vi "rsidr_core_global.vi"() -> ()   [LabVIEW 2015, in "Rohde&Schwarz CMXP GPRF.lvlib"] (continued)
 All", "Data Type"=6, "Command"="FETC:GPRF:MEAS{instance}:POW:STAT:ALL?", "Access"=0, "Range Table"="", "Read Callback"="", "Write Callback"="", "Supported Models"="", "Instrument Options"="", "Flags"=0, "Help"="Queries the main measurement state and the measurement substates. Both measurement substates are relevant for running measurements only.\n\nAvailable Repeated Capabilities:\ninstance: i0, i1, i2, i3, i4, i5, i6, i7, i8, i9, i10, i11, i12, i13, i14, i15, i16, i17, i18, i19, i20, i21, i22, i23, i24, i25, i26, i27, i28, i29, i30, i31, i32\r\n\nRemote-control command(s):\nFETCh:GPRF:MEAS<i>:POWer:STATe:ALL?"}, {"Level"=3, "Class Only"=FALSE, "Identifier"="RSCMXPGPRF_ATTR_POWER_MEASUREMENT_ELAPSED_INTERVALS", "Descriptive Name"="Power Measurement Elapsed Intervals", "Data Type"=6, "Command"="FETC:GPRF:MEAS{instance}:POW:EST?", "Access"=0, "Range Table"="", "Read Callback"="", "Write Callback"="", "Supported Models"="", "Instrument Options"="", "Flags"=0, "Help"="Returns the reliability indicator and the number of elapsed measurement intervals.\n\nAvailable Repeated Capabilities:\ninstance: i0, i1, i2, i3, i4, i5, i6, i7, i8, i9, i10, i11, i12, i13, i14, i15, i16, i17, i18, i19, i20, i21, i22, i23, i24, i25, i26, i27, i28, i29, i30, i31, i32\r\n\nRemote-control command(s):\nFETCh:GPRF:MEAS<i>:POWer:ESTatistics?"}, {"Level"=2, "Class Only"=TRUE, "Identifier"="", "Descriptive Name"="Results", "Data Type"=0, "Command"="", "Access"=0, "Range Table"="", "Read Callback"="", "Write Callback"="", "Supported Models"="", "Instrument Options"="", "Flags"=0, "Help"="Power measurement results."}, {"Level"=3, "Class Only"=FALSE, "Identifier"="RSCMXPGPRF_ATTR_POWER_MEASUREMENT_POWER_CURRENT", "Descriptive Name"="Power Measurement Power Current", "Data Type"=6, "Command"="CALC:GPRF:MEAS{instance}:POW:CURR?", "Access"=0, "Range Table"="", "Read Callback"="", "Write Callback"="", "Supported Models"="", "Instrument Options"="", "Flags"=0, "Help"="Returns results for the Power mode.\n\nAvailable Repeated Capabilities:\ninstance: i0, i1, i2, i3, i4, i5, i6, i7, i8, i9, i10, i11, i12, i13, i14, i15, i16, i17, i18, i19, i20, i21, i22, i23, i24, i25, i26, i27, i28, i29, i30, i31, i32\r\n\nRemote-control command(s):\nCALCulate:GPRF:MEAS<i>:POWer:CURRent?"}, {"Level"=3, "Class Only"=FALSE, "Identifier"="RSCMXPGPRF_ATTR_FETCH_POWER_MEASUREMENT_POWER_CURRENT", "Descriptive Name"="Fetch Power Measurement Power Current", "Data Type"=6, "Command"="FETC:GPRF:MEAS{instance}:POW:CURR?", "Access"=0, "Range Table"="", "Read Callback"="", "Write Callback"="", "Supported Models"="", "Instrument Options"="", "Flags"=0, "Help"="Returns results for the Power mode.\n\nAvailable Repeated Capabilities:\ninstance: i0, i1, i2, i3, i4, i5, i6, i7, i8, i9, i10, i11, i12, i13, i14, i15, i16, i17, i18, i19, i20, i21, i22, i23, i24, i25, i26, i27, i28, i29, i30, i31, i32\r\n\nRemote-control command(s):\nFETCh:GPRF:MEAS<i>:POWer:CURRent?"}, {"Level"=3, "Class Only"=FALSE, "Identifier"="RSCMXPGPRF_ATTR_READ_POWER_MEASUREMENT_POWER_CURRENT", "Descriptive Name"="Read Power Measurement Power Current", "Data Type"=6, "Command"="READ:GPRF:MEAS{instance}:POW:CURR?", "Access"=0, "Range Table"="", "Read Callback"="", "Write Callback"="", "Supported Models"="", "Instrument Options"="", "Flags"=0, "Help"="Returns results for the Power mode.\n\nAvailable Repeated Capabilities:\ninstance: i0, i1, i2, i3, i4, i5, i6, i7, i8, i9, i10, i11, i12, i13, i14, i15, i16, i17, i18, i19, i20, i21, i22, i23, i24, i25, i26, i27, i28, i29, i30, i31, i32\r\n\nRemote-control command(s):\nREAD:GPRF:MEAS<i>:POWer:CURRent?"}, {"Level"=3, "Class Only"=FALSE, "Identifier"="RSCMXPGPRF_ATTR_READ_POWER_MEASUREMENT_POWER_AVERAGE", "Descriptive Name"="Read Power Measurement Power Average", "Data Type"=6, "Command"="READ:GPRF:MEAS{instance}:POW:AVER?", "Access"=0, "Range Table"="", "Read Callback"="", "Write Callback"="", "Supported Models"="", "Instrument Options"="", "Flags"=0, "Help"="Returns results for the Power mode.\n\nAvailable Repeated Capabilities:\ninstance: i0, i1, i2, i3, i4, i5, i6, i7, i8, i9, i10, i11, i12, i13, i14, i15, i16, i17, i18, i19, i20, i21, i22, i23, i24, i25, i26, i27, i28, i29, i30, i31, i32\r\n\nRemote-control command(s):\nREAD:GPRF:MEAS<i>:POWer:AVERage?"}, {"Level"=3, "Class Only"=FALSE, "Identifier"="RSCMXPGPRF_ATTR_READ_POWER_MEASUREMENT_MINIMUM_CURRENT", "Descriptive Name"="Read Power Measurement Minimum Current", "Data Type"=6, "Command"="READ:GPRF:MEAS{instance}:POW:MIN:CURR?", "Access"=0, "Range Table"="", "Read Callback"="", "Write Callback"="", "Supported Models"="", "Instrument Options"="", "Flags"=0, "Help"="Returns results for the Power mode.\n\nAvailable Repeated Capabilities:\ninstance: i0, i1, i2, i3, i4, i5, i6, i7, i8, i9, i10, i11, i12, i13, i14, i15, i16, i17, i18, i19, i20, i21, i22, i23, i24, i25, i26, i27, i28, i29, i30, i31, i32\r\n\nRemote-control command(s):\nREAD:GPRF:MEAS<i>:POWer:MINimum:CURRent?"}, {"Level"=3, "Class Only"=FALSE, "Identifier"="RSCMXPGPRF_ATTR_READ_POWER_MEASUREMENT_MAXIMUM_CURRENT", "Descriptive Name"="Read Power Measurement Maximum Current", "Data Type"=6, "Command"="READ:GPRF:MEAS{instance}:POW:MAX:CURR?", "Access"=0, "Range Table"="", "Read Callback"="", "Write Callback"="", "Supported Models"="", "Instrument Options"="", "Flags"=0, "Help"="Returns results for the Power mode.\n\nAvailable Repeated Capabilities:\ninstance: i0, i1, i2, i3, i4, i5, i6, i7, i8, i9, i10, i11, i12, i13, i14, i15, i16, i17, i18, i19, i20, i21, i22, i23, i24, i25, i26, i27, i28, i29, i30, i31, i32\r\n\nRemote-control command(s):\nREAD:GPRF:MEAS<i>:POWer:MAXimum:CURRent?"}, {"Level"=3, "Class Only"=FALSE, "Identifier"="RSCMXPGPRF_ATTR_READ_POWER_MEASUREMENT_MINIMUM_PEAK", "Descriptive Name"="Read Power Measurement Minimum Peak", "Data Type"=6, "Command"="READ:GPRF:MEAS{instance}:POW:PEAK:MIN?", "Access"=0, "Range Table"="", "Read Callback"="", "Write Callback"="", "Supported Models"="", "Instrument Options"="", "Flags"=0, "Help"="Returns results for the Power mode.\n\nAvailable Repeated Capabilities:\ninstance: i0, i1, i2, i3, i4, i5, i6, i7, i8, i9, i10, i11, i12, i13, i14, i15, i16, i17, i18, i19, i20, i21, i22, i23, i24, i25, i26, i27, i28, i29, i30, i31, i32\r\n\nRemote-control command(s):\nREAD:GPRF:MEAS<i>:POWer:PEAK:MINimum?"}, {"Level"=3, "Class Only"=FALSE, "Identifier"="RSCMXPGPRF_ATTR_READ_POWER_MEASUREMENT_MAXIMUM_PEAK", "Descriptive Name"="Read Power Measurement Maximum Peak", "Data Type"=6, "Command"="READ:GPRF:MEAS{instance}:POW:PEAK:MAX?", "Access"=0, "Range Table"="", "Read Callback"="", "Write Callback"="", "Supported Models"="", "Instrument Options"="", "Flags"=0, "Help"="Returns results for the Power mode.\n\nAvailable Repeated Capabilities:\ninstance: i0, i1, i2, i3, i4, i5, i6, i7, i8, i9, i10, i11, i12, i13, i14, i15, i16, i17, i18, i19, i20, i21, i22, i23, i24, i25, i26, i27, i28, i29, i30, i31, i32\r\n\nRemote-control command(s):\nREAD:GPRF:MEAS<i>:POWer:PEAK:MAXimum?"}, {"Level"=3, "Class Only"=FALSE, "Identifier"="RSCMXPGPRF_ATTR_FETCH_POWER_MEASUREMENT_MINIMUM_CURRENT", "Descriptive Name"="Fetch Power Measurement Minimum Current", "Data Type"=6, "Command"="FETC:GPRF:MEAS{instance}:POW:MIN:CURR?", "Access"=0, "Range Table"="", "Read Callback"="", "Write Callback"="", "Supported Models"="", "Instrument Options"="", "Flags"=0, "Help"="Returns results for the Power mode.\n\nAvailable Repeated Capabilities:\ninstance: i0, i1, i2, i3, i4, i5, i6, i7, i8, i9, i10, i11, i12, i13, i14, i15, i16, i17, i18, i19, i20, i21, i22, i23, i24, i25, i26, i27, i28, i29, i30, i31, i32\r\n\nRemote-control command(s):\nFETCh:GPRF:MEAS<i>:POWer:MINimum:CURRent?"}, {"Level"=3, "Class Only"=FALSE, "Identifier"="RSCMXPGPRF_ATTR_FETCH_POWER_MEASUREMENT_MAXIMUM_CURRENT", "Descriptive Name"="Fetch Power Measurement Maximum Current", "Data Type"=6, "Command"="FETC:GPRF:MEAS{instance}:POW:MAX:CURR?", "Access"=0, "Range Table"="", "Read Callback"="", "Write Callback"="", "Supported Models"="", "Instrument Options"="", "Flags"=0, "Help"="Returns results for the Power mode.\n\nAvailable Repeated Capabilities:\ninstance: i0, i1, i2, i3, i4, i5, i6, i7, i8, i9, i10, i11, i12, i13, i14, i15, i16, i17, i18, i19, i20, i21, i22, i23, i24, i25, i26, i27, i28, i29, i30, i31, i32\r\n\nRemote-control command(s):\nFETCh:GPRF:MEAS<i>:POWer:MAXimum:CURRent?"}, {"Level"=3, "Class Only"=FALSE, "Identifier"="RSCMXPGPRF_ATTR_FETCH_POWER_MEASUREMENT_AVERAGE", "Descriptive Name"="Fetch Power Measurement Average", "Data Type"=6, "Command"="FETC:GPRF:MEAS{instance}:POW:AVER?", "Access"=0, "Range Table"="", "Read Callback"="", "Write Callback"="", "Supported Models"="", "Instrument Options"="", "Flags"=0, "Help"="Returns results for the Power mode.\n\nAvailable Repeated Capabilities:\ninstance: i0, i1, i2, i3, i4, i5, i6, i7, i8, i9, i10, i11, i12, i13, i14, i15, i16, i17, i18, i19, i20, i21, i22, i23, i24, i25, i26, i27, i28, i29, i30, i31, i32\r\n\nRemote-control command(s):\nFETCh:GPRF:MEAS<i>:POWer:AVERage?"}, {"Level"=3, "Class Only"=FALSE, "Identifier"="RSCMXPGPRF_ATTR_FETCH_POWER_MEASUREMENT_MINIMUM_PEAK", "Descriptive Name"="Fetch Power Measurement Minimum Peak", "Data Type"=6, "Command"="FETC:GPRF:MEAS{instance}:POW:PEAK:MIN?", "Access"=0, "Range Table"="", "Read Callback"="", "Write Callback"="", "Supported Models"="", "Instrument Options"="", "Flags"=0, "Help"="Returns results for the Power mode.\n\nAvailable Repeated Capabilities:\ninstance: i0, i1, i2, i3, i4, i5, i6, i7, i8, i9, i10, i11, i12, i13, i14, i15, i16, i17, i18, i19, i20, i21, i22, i23, i24, i25, i26, i27, i28, i29, i30, i31, i32\r\n\nRemote-control command(s):\nFETCh:GPRF:MEAS<i>:POWer:PEAK:MINimum?"}, {"Level"=3, "Class Only"=FALSE, "Identifier"="RSCMXPGPRF_ATTR_FETCH_POWER_MEASUREMENT_MAXIMUM_PEAK", "Descriptive Name"="Fetch Power Measurement Maximum Peak", "Data Type"=6, "Command"="FETC:GPRF:MEAS{instance}:POW:PEAK:MAX?", "Access"=0, "Range Table"="", "Read Callback"="", "Write Callback"="", "Supported Models"="", "Instrument Options"="", "Flags"=0, "Help"="Returns results for the Power mode.\n\nAvailable Repeated Capabilities:\ninstance: i0, i1, i2, i3, i4, i5, i6, i7, i8, i9, i10, i11, i12, i13, i14, i15, i16, i17, i18, i19, i20, i21, i22, i23, i24, i25, i26, i27, i28, i29, i30, i31, i32\r\n\nRemote-control command(s):\nFETCh:GPRF:MEAS<i>:POWer:PEAK:MAXimum?"}, {"Level"=3, "Class Only"=FALSE, "Identifier"="RSCMXPGPRF_ATTR_POWER_MEASUREMENT_LIMIT_CHECK_RESULT_MINIMUM_CURRENT", "Descriptive Name"="Power Measurement Limit Check Result Minimum Current", "Data Type"=6, "Command"="CALC:GPRF:MEAS{instance}:POW:MIN:CURR?", "Access"=0, "Range Table"="", "Read Callback"="", "Write Callback"="", "Supported Models"="", "Instrument Options"="", "Flags"=0, "Help"="Returns results for the Power mode.\n\nAvailable Repeated Capabilities:\ninstance: i0, i1, i2, i3, i4, i5, i6, i7, i8, i9, i10, i11, i12, i13, i14, i15, i16, i17, i18, i19, i20, i21, i22, i23, i24, i25, i26, i27, i28, i29, i30, i31, i32\r\n\nRemote-control command(s):\nCALCulate:GPRF:MEAS<i>:POWer:MINimum:CURRent?"}, {"Level"=3, "Class Only"=FALSE, "Identifier"="RSCMXPGPRF_ATTR_POWER_MEASUREMENT_LIMIT_CHECK_RESULT_MAXIMUM_CURRENT", "Descriptive Name"="Power Measurement Limit Check Result Maximum Current", "Data Type"=6, "Command"="CALC:GPRF:MEAS{instance}:POW:MAX:CURR?", "Access"=0, "Range Table"="", "Read Callback"="", "Write Callback"="", "Supported Models"="", "Instrument Options"="", "Flags"=0, "Help"="Returns results for the Power mode.\n\nAvailable Repeated Capabilities:\ninstance: i0, i1, i2, i3, i4, i5, i6, i7, i8, i9, i10, i11, i12, i13, i14, i15, i16, i17, i18, i19, i20, i21, i22, i23, i24, i25, i26, i27, i28, i29, i30, i31, i32\r\n\nRemote-control command(s):\nCALCulate:GPRF:MEAS<i>:POWer:MAXimum:CURRent?"}, {"Level"=3, "Class Only"=FALSE, "Identifier"="RSCMXPGPRF_ATTR_POWER_MEASUREMENT_LIMIT_CHECK_RESULT_AVERAGE", "Descriptive Name"="Power Measurement Limit Check Result Average", "Data Type"=6, "Command"="CALC:GPRF:MEAS{instance}:POW:AVER?", "Access"=0, "Range Table"="", "Read Callback"="", "Write Callback"="", "Supported Models"="", "Instrument Options"="", "Flags"=0, "Help"="Returns results for the Power mode.\n\nAvailable Repeated Capabilities:\ninstance: i0, i1, i2, i3, i4, i5, i6, i7, i8, i9, i10, i11, i12, i13, i14, i15, i16, i17, i18, i19, i20, i21, i22, i23, i24, i25, i26, i27, i28, i29, i30, i31, i32\r\n\nRemote-control command(s):\nCALCulate:GPRF:MEAS<i>:POWer:AVERage?"}, {"Level"=3, "Class Only"=FALSE, "Identifier"="RSCMXPGPRF_ATTR_POWER_MEASUREMENT_LIMIT_CHECK_RESULT_PEAK_MINIMUM", "Descriptive Name"="Power Measurement Limit Check Result Peak Minimum", "Data Type"=6, "Command"="CALC:GPRF:MEAS{instance}:POW:PEAK:MIN?", "Access"=0, "Range Table"="", "Read Callback"="", "Write Callback"="", "Supported Models"="", "Instrument Options"="", "Flags"=0, "Help"="Returns results for the Power mode.\n\nAvailable Repeated Capabilities:\ninstance: i0, i1, i2, i3, i4, i5, i6, i7, i8, i9, i10, i11, i12, i13, i14, i15, i16, i17, i18, i19, i20, i21, i22, i23, i24, i25, i26, i27, i28, i29, i30, i31, i32\r\n\nRemote-control command(s):\nCALCulate:GPRF:MEAS<i>:POWer:PEAK:MINimum?"}, {"Level"=3, "Class Only"=FALSE, "Identifier"="RSCMXPGPRF_ATTR_POWER_MEASUREMENT_LIMIT_CHECK_RESULT_PEAK_MAXIMUM", "Descriptive Name"="Power Measurement Limit Check Result Peak Maximum", "Data Type"=6, "Command"="CALC:GPRF:MEAS{instance}:POW:PEAK:MAX?", "Access"=0, "Range Table"="", "Read Callback"="", "Write Callback"="", "Supported Models"="", "Instrument Options"="", "Flags"=0, "Help"="Returns results for the Power mode.\n\nAvailable Repeated Capabilities:\ninstance: i0, i1, i2, i3, i4, i5, i6, i7, i8, i9, i10, i11, i12, i13, i14, i15, i16, i17, i18, i19, i20, i21, i22, i23, i24, i25, i26, i27, i28, i29, i30, i31, i32\r\n\nRemote-control command(s):\nCALCulate:GPRF:MEAS<i>:POWer:PEAK:MAXimum?"}, {"Level"=3, "Class Only"=FALSE, "Identifier"="RSCMXPGPRF_ATTR_READ_POWER_MEASUREMENT_STANDARD_DEVIATION", "Descriptive Name"="Read Power Measurement Standard Deviation", "Data Type"=6, "Command"="READ:GPRF:MEAS{instance}:POW:SDEV?", "Access"=0, "Range Table"="", "Read Callback"="", "Write Callback"="", "Supported Models"="", "Instrument Options"="", "Flags"=0, "Help"="Returns results for the Power mode.\n\nAvailable Repeated Capabilities:\ninstance: i0, i1, i2, i3, i4, i5, i6, i7, i8, i9, i10, i11, i12, i13, i14, i15, i16, i17, i18, i19, i20, i21, i22, i23, i24, i25, i26, i27, i28, i29, i30, i31, i32\r\n\nRemote-control command(s):\nREAD:GPRF:MEAS<i>:POWer:SDEViation?"}, {"Level"=3, "Class Only"=FALSE, "Identifier"="RSCMXPGPRF_ATTR_POWER_MEASUREMENT_STANDARD_DEVIATION", "Descriptive Name"="Power Measurement Standard Deviation", "Data Type"=6, "Command"="CALC:GPRF:MEAS{instance}:POW:SDEV?", "Access"=0, "Range Table"="", "Read Callback"="", "Write Callback"="", "Supported Models"="", "Instrument Options"="", "Flags"=0, "Help"="Returns results for the Power mode.\n\nAvailable Repeated Capabilities:\ninstance: i0, i1, i2, i3, i4, i5, i6, i7, i8, i9, i10, i11, i12, i13, i14, i15, i16, i17, i18, i19, i20, i21, i22, i23, i24, i25, i26, i27, i28, i29, i30, i31, i32\r\n\nRemote-control command(s):\nCALCulate:GPRF:MEAS<i>:POWer:SDEViation?"}, {"Level"=3, "Class Only"=FALSE, "Identifier"="RSCMXPGPRF_ATTR_HIDDEN_READ_POWER_MEASUREMENT_LIST_CURRENT", "Descriptive Name"="Read Power Measurement List Current", "Data Type"=6, "Command"="READ:GPRF:MEAS{instance}:POW:LIST:CURR?", "Access"=0, "Range Table"="", "Read Callback"="", "Write Callback"="", "Supported Models"="", "Instrument Options"="", "Flags"=8, "Help"="Returns power results for segment <ListIndex>, see Results in List Mode.\n\nAvailable Repeated Capabilities:\ninstance: i0, i1, i2, i3, i4, i5, i6, i7, i8, i9, i10, i11, i12, i13, i14, i15, i16, i17, i18, i19, i20, i21, i22, i23, i24, i25, i26, i27, i28, i29, i30, i31, i32\r\n\nRemote-control command(s):\nREAD:GPRF:MEAS<i>:POWer:LIST:CURRent?"}, {"Level"=3, "Class Only"=FALSE, "Identifier"="RSCMXPGPRF_ATTR_HIDDEN_READ_POWER_MEASUREMENT_LIST_MAXIMUM_CURRENT", "Descriptive Name"="Read Power Measurement List Maximum Current", "Data Type"=6, "Command"="READ:GPRF:MEAS{instance}:POW:LIST:MAX:CURR?", "Access"=0, "Range Table"="", "Read Callback"="", "Write Callback"="", "Supported Models"="", "Instrument Options"="", "Flags"=8, "Help"="Returns power results for segment <ListIndex>, see Results in List Mode.\n\nAvailable Repeated Capabilities:\ninstance: i0, i1, i2, i3, i4, i5, i6, i7, i8, i9, i10, i11, i12, i13, i14, i15, i16, i17, i18, i19, i20, i21, i22, i23, i24, i25, i26, i27, i28, i29, i30, i31, i32\r\n\nRemote-control command(s):\nREAD:GPRF:MEAS<i>:POWer:LIST:MAXimum:CURRent?"}, {"Level"=3, "Class Only"=FALSE, "Identifier"="RSCMXPGPRF_ATTR_HIDDEN_READ_POWER_MEASUREMENT_LIST_MINIMUM_CURRENT", "Descriptive Name"="Read Power Measurement List Minimum Current", "Data Type"=6, "Command"="READ:GPRF:MEAS{instance}:POW:LIST:MIN:CURR?", "Access"=0, "Range Table"="", "Read Callback"="", "Write Callback"="", "Supported Models"="", "Instrument Options"="", "Flags"=8, "Help"="Returns power results for segment <ListIndex>, see Results in List Mode.\n\nAvailable Repeated Capabilities:\ninstance: i0, i1, i2, i3, i4, i5, i6, i7, i8, i9, i10, i11, i12, i13, i14, i15, i16, i17, i18, i19, i20, i21, i22, i23, i24, i25, i26, i27, i28, i29, i30, i31, i32\r\n\nRemote-control command(s):\nREAD:GPRF:MEAS<i>:POWer:LIST:MINimum:CURRent?"}, {"Level"=3, "Class Only"=FALSE, "Identifier"="RSCMXPGPRF_ATTR_HIDDEN_READ_POWER_MEASUREMENT_LIST_AVERAGE", "Descriptive Name"="Read Power Measurement List Average", "Data Type"=6, "Command"="READ:GPRF:MEAS{instance}:POW:LIST:AVER?", "Access"=0, "Range Table"="", "Read Callback"="", "Write Callback"="", "Supported Models"="", "Instrument Options"="", "Flags"=8, "Help"="Returns power results for segment <ListIndex>, see Results in List Mode.\n\nAvailable Repeated Capabilities:\ninstance: i0, i1, i2, i3, i4, i5, i6, i7, i8, i9, i10, i11, i12, i13, i14, i15, i16, i17, i18, i19, i20, i21, i22, i23, i24, i25, i26, i27, i28, i29, i30, i31, i32\r\n\nRemote-control command(s):\nREAD:GPRF:MEAS<i>:POWer:LIST:AVERage?"}, {"Level"=3, "Class Only"=FALSE, "Identifier"="RSCMXPGPRF_ATTR_HIDDEN_READ_POWER_MEASUREMENT_LIST_MAXIMUM_PEAK", "Descriptive Name"="Read Power Measurement List Maximum Peak", "Data Type"=6, "Command"="READ:GPRF:MEAS{instance}:POW:LIST:PEAK:MAX?", "Access"=0, "Range Table"="", "Read Callback"="", "Write Callback"="", "Supported Models"="", "Instrument Options"="", "Flags"=8, "Help"="Returns power results for segment <ListIndex>, see Results in List Mode.\n\nAvailable Repeated Capabilities:\ninstance: i0, i1, i2, i3, i4, i5, i6, i7, i8, i9, i10, i11, i12, i13, i14, i15, i16, i17, i18, i19, i20, i21, i22, i23, i24, i25, i26, i27, i28, i29, i30, i31, i32\r\n\nRemote-control command(s):\nREAD:GPRF:MEAS<i>:POWer:LIST:PEAK:MAXimum?"}, {"Level"=3, "Class Only"=FALSE, "Identifier"="RSCMXPGPRF_ATTR_HIDDEN_READ_POWER_MEASUREMENT_LIST_MINIMUM_PEAK", "Descriptive Name"="Read Power Measurement List Minimum Peak", "Data Type"=6, "Command"="READ:GPRF:MEAS{instance}:POW:LIST:PEAK:MIN?", "Access"=0, "Range Table"="", "Read Callback"="", "Write Callback"="", "Supported Models"="", "Instrument Options"="", "Flags"=8, "Help"="Returns power results for segment <ListIndex>, see Results in List Mode.\n\nAvailable Repeated Capabilities:\ninstance: i0, i1, i2, i3, i4, i5, i6, i7, i8, i9, i10, i11, i12, i13, i14, i15, i16, i17, i18, i19, i20, i21, i22, i23, i24, i25, i26, i27, i28, i29, i30, i31, i32\r\n\nRemote-control command(s):\nREAD:GPRF:MEAS<i>:POWer:LIST:PEAK:MINimum?"}, {"Level"=3, "Class Only"=FALSE, "Identifier"="RSCMXPGPRF_ATTR_HIDDEN_FETCH_POWER_MEASUREMENT_LIST_CURRENT", "Descriptive Name"="Fetch Power Measurement List Current", "Data Type"=6, "Command"="FETC:GPRF:MEAS{instance}:POW:LIST:CURR?", "Access"=0, "Range Table"="", "Read Callback"="", "Write Callback"="", "Supported Models"="", "Instrument Options"="", "Flags"=8, "Help"="Returns power results for segment <ListIndex>, see Results in List Mode.\n\nAvailable Repeated Capabilities:\ninstance: i0, i1, i2, i3, i4, i5, i6, i7, i8, i9, i10, i11, i12, i13, i14, i15, i16, i17, i18, i19, i20, i21, i22, i23, i24, i25, i26, i27, i28, i29, i30, i31, i32\r\n\nRemote-control command(s):\nFETCh:GPRF:MEAS<i>:POWer:LIST:CURRent?"}, {"Level"=3, "Class Only"=FALSE, "Identifier"="RSCMXPGPRF_ATTR_HIDDEN_FETCH_POWER_MEASUREMENT_LIST_MAXIMUM_CURRENT", "Descriptive Name"="Fetch Power Measurement List Maximum Current", "Data Type"=2, "Command"="FETC:GPRF:MEAS{instance}:POW:LIST:MAX:CURR?", "Access"=0, "Range Table"="", "Read Callback"="", "Write Callback"="", "Supported Models"="", "Instrument Options"="", "Flags"=8, "Help"="Returns power results for segment <ListIndex>, see Results in List Mode.\n\nAvailable Repeated Capabilities:\ninstance: i0, i1, i2, i3, i4, i5, i6, i7, i8, i9, i10, i11, i12, i13, i14, i15, i16, i17, i18, i19, i20, i21, i22, i23, i24, i25, i26, i27, i28, i29, i30, i31, i32\r\n\nRemote-control command(s):\nFETCh:GPRF:MEAS<i>:POWer:LIST:MAXimum:CURRent?"}, {"Level"=3, "Class Only"=FALSE, "Identifier"="RSCMXPGPRF_ATTR_HIDDEN_FETCH_POWER_MEASUREMENT_LIST_MINIMUM_CURRENT", "Descriptive Name"="Fetch Power Measurement List Minimum Current", "Data Type"=6, "Command"="FETC:GPRF:MEAS{instance}:POW:LIST:MIN:CURR?", "Access"=0, "Range Table"="", "Read Callback"="", "Write Callback"="", "Supported Models"="", "Instrument Options"="", "Flags"=8, "Help"="Returns power results for segment <ListIndex>, see Results in List Mode.\n\nAvailable Repeated Capabilities:\ninstance: i0, i1, i2, i3, i4, i5, i6, i7, i8, i9, i10, i11, i12, i13, i14, i15, i16, i17, i18, i19, i20, i21, i22, i23, i24, i25, i26, i27, i28, i29, i30, i31, i32\r\n\nRemote-control command(s):\nFETCh:GPRF:MEAS<i>:POWer:LIST:MINimum:CURRent?"}, {"Level"=3, "Class Only"=FALSE, "Identifier"="RSCMXPGPRF_ATTR_HIDDEN_FETCH_POWER_MEASUREMENT_LIST_AVERAGE", "Descriptive Name"="Fetch Power Measurement List Average", "Data Type"=6, "Command"="FETC:GPRF:MEAS{instance}:POW:LIST:AVER?", "Access"=0, "Range Table"="", "Read Callback"="", "Write Callback"="", "Supported Models"="", "Instrument Options"="", "Flags"=8, "Help"="Returns power results for segment <ListIndex>, see Results in List Mode.\n\nAvailable Repeated Capabilities:\ninstance: i0, i1, i2, i3, i4, i5, i6, i7, i8, i9, i10, i11, i12, i13, i14, i15, i16, i17, i18, i19, i20, i21, i22, i23, i24, i25, i26, i27, i28, i29, i30, i31, i32\r\n\nRemote-control command(s):\nFETCh:GPRF:MEAS<i>:POWer:LIST:AVERage?"}, {"Level"=3, "Class Only"=FALSE, "Identifier"="RSCMXPGPRF_ATTR_HIDDEN_FETCH_POWER_MEASUREMENT_LIST_MAXIMUM_PEAK", "Descriptive Name"="Fetch Power Measurement List Maximum Peak", "Data Type"=6, "Command"="FETC:GPRF:MEAS{instance}:POW:LIST:PEAK:MAX?", "Access"=0, "Range Table"="", "Read Callback"="", "Write Callback"="", "Supported Models"="", "Instrument Options"="", "Flags"=8, "Help"="Returns power results for segment <ListIndex>, see Results in List Mode.\n\nAvailable Repeated Capabilities:\ninstance: i0, i1, i2, i3, i4, i5, i6, i7, i8, i9, i10, i11, i12, i13, i14, i15, i16, i17, i18, i19, i20, i21, i22, i23, i24, i25, i26, i27, i28, i29, i30, i31, i32\r\n\nRemote-control command(s):\nFETCh:GPRF:MEAS<i>:POWer:LIST:PEAK:MAXimum?"}, {"Level"=3, "Class Only"=FALSE, "Identifier"="RSCMXPGPRF_ATTR_HIDDEN_FETCH_POWER_MEASUREMENT_LIST_MINIMUM_PEAK", "Descriptive Name"="Fetch Power Measurement List Minimum Peak", "Data Type"=6, "Command"="FETC:GPRF:MEAS{instance}:POW:LIST:PEAK:MIN?", "Access"=0, "Range Table"="", "Read Callback"="", "Write Callback"="", "Supported Models"="", "Instrument Options"="", "Flags"=8, "Help"="Returns power results for segment <ListIndex>, see Results in List Mode.\n\nAvailable Repeated Capabilities:\ninstance: i0, i1, i2, i3, i4, i5, i6, i7, i8, i9, i10, i11, i12, i13, i14, i15, i16, i17, i18, i19, i20, i21, i22, i23, i24, i25, i26, i27, i28, i29, i30, i31, i32\r\n\nRemote-control command(s):\nFETCh:GPRF:MEAS<i>:POWer:LIST:PEAK:MINimum?"}, {"Level"=3, "Class Only"=FALSE, "Identifier"="RSCMXPGPRF_ATTR_READ_POWER_MEASUREMENT_ERROR_CODES_LIST_CURRENT", "Descriptive Name"="Read Power Measurement Error Codes List Current", "Data Type"=6, "Command"="READ:GPRF:MEAS{instance}:POW:SDEV?", "Access"=0, "Range Table"="", "Read Callback"="", "Write Callback"="", "Supported Models"="", "Instrument Options"="", "Flags"=0, "Help"="Returns power results for all segments, see Results in List Mode.\n\nAvailable Repeated Capabilities:\ninstance: i0, i1, i2, i3, i4, i5, i6, i7, i8, i9, i10, i11, i12, i13, i14, i15, i16, i17, i18, i19, i20, i21, i22, i23, i24, i25, i26, i27, i28, i29, i30, i31, i32\r\n\nRemote-control command(s):\nREAD:GPRF:MEAS<i>:POWer:SDEViation?"}, {"Level"=3, "Class Only"=FALSE, "Identifier"="RSCMXPGPRF_ATTR_HIDDEN_POWER_MEASUREMENT_LIMIT_CHECK_RESULT_LIST_CURRENT", "Descriptive Name"="Power Measurement Limit Check Result List Current", "Data Type"=6, "Command"="CALC:GPRF:MEAS{instance}:POW:LIST:CURR?", "Access"=0, "Range Table"="", "Read Callback"="", "Write Callback"="", "Supported Models"="", "Instrument Options"="", "Flags"=8, "Help"="Returns power results for segment <ListIndex>, see Results in List Mode.\n\nAvailable Repeated Capabilities:\ninstance: i0, i1, i2, i3, i4, i5, i6, i7, i8, i9, i10, i11, i12, i13, i14, i15, i16, i17, i18, i19, i20, i21, i22, i23, i24, i25, i26, i27, i28, i29, i30, i31, i32\r\n\nRemote-control command(s):\nCALCulate:GPRF:MEAS<i>:POWer:LIST:CURRent?"}, {"Level"=3, "Class Only"=FALSE, "Identifier"="RSCMXPGPRF_ATTR_HIDDEN_POWER_MEASUREMENT_LIMIT_CHECK_RESULT_LIST_MAXIMUM_CURRENT", "Descriptive Name"="Power Measurement Limit Check Result List Maximum Current", "Data Type"=6, "Command"="CALC:GPRF:MEAS{instance}:POW:LIST:MAX:CURR?", "Access"=0, "Range Table"="", "Read Callback"="", "Write Callback"="", "Supported Models"="", "Instrument Options"="", "Flags"=8, "Help"="Returns power results for segment <ListIndex>, see Results in List Mode.\n\nAvailable Repeated Capabilities:\ninstance: i0, i1, i2, i3, i4, i5, i6, i7, i8, i9, i10, i11, i12, i13, i14, i15, i16, i17, i18, i19, i20, i21, i22, i23, i24, i25, i26, i27, i28, i29, i30, i31, i32\r\n\nRemote-control command(s):\nCALCulate:GPRF:MEAS<i>:POWer:LIST:MAXimum:CURRent?"}, {"Level"=3, "Class Only"=FALSE, "Identifier"="RSCMXPGPRF_ATTR_HIDDEN_POWER_MEASUREMENT_LIMIT_CHECK_RESULT_LIST_MINIMUM_CURRENT", "Descriptive Name"="Power Measurement Limit Check Result List Minimum Current", "Data Type"=6, "Command"="CALC:GPRF:MEAS{instance}:POW:LIST:MIN:CURR?", "Access"=0, "Range Table"="", "Read Callback"="", "Write Callback"="", "Supported Models"="", "Instrument Options"="", "Flags"=8, "Help"="Returns power results for segment <ListIndex>, see Results in List Mode.\n\nAvailable Repeated Capabilities:\ninstance: i0, i1, i2, i3, i4, i5, i6, i7, i8, i9, i10, i11, i12, i13, i14, i15, i16, i17, i18, i19, i20, i21, i22, i23, i24, i25, i26, i27, i28, i29, i30, i31, i32\r\n\nRemote-control command(s):\nCALCulate:GPRF:MEAS<i>:POWer:LIST:MINimum:CURRent?"}, {"Level"=3, "Class Only"=FALSE, "Identifier"="RSCMXPGPRF_ATTR_HIDDEN_POWER_MEASUREMENT_LIMIT_CHECK_RESULT_LIST_AVERAGE", "Descriptive Name"="Power Measurement Limit Check Result List Average", "Data Type"=6, "Command"="CALC:GPRF:MEAS{instance}:POW:LIST:AVER?", "Access"=0, "Range Table"="", "Read Callback"="", "Write Callback"="", "Supported Models"="", "Instrument Options"="", "Flags"=8, "Help"="Returns power results for segment <ListIndex>, see Results in List Mode.\n\nAvailable Repeated Capabilities:\ninstance: i0, i1, i2, i3, i4, i5, i6, i7, i8, i9, i10, i11, i12, i13, i14, i15, i16, i17, i18, i19, i20, i21, i22, i23, i24, i25, i26, i27, i28, i29, i30, i31, i32\r\n\nRemote-control command(s):\nCALCulate:GPRF:MEAS<i>:POWer:LIST:AVERage?"}, {"Level"=3, "Class Only"=FALSE, "Identifier"="RSCMXPGPRF_ATTR_HIDDEN_POWER_MEASUREMENT_LIMIT_CHECK_RESULT_LIST_MAXIMUM_PEAK", "Descriptive Name"="Power Measurement Limit Check Result List Maximum Peak", "Data Type"=6, "Command"="CALC:GPRF:MEAS{instance}:POW:LIST:PEAK:MAX?", "Access"=0, "Range Table"="", "Read Callback"="", "Write Callback"="", "Supported Models"="", "Instrument Options"="", "Flags"=8, "Help"="Returns power results for segment <ListIndex>, see Results in List Mode.\n\nAvailable Repeated Capabilities:\ninstance: i0, i1, i2, i3, i4, i5, i6, i7, i8, i9, i10, i11, i12, i13, i14, i15, i16, i17, i18, i19, i20, i21, i22, i23, i24, i25, i26, i27, i28, i29, i30, i31, i32\r\n\nRemote-control command(s):\nCALCulate:GPRF:MEAS<i>:POWer:LIST:PEAK:MAXimum?"}, {"Level"=3, "Class Only"=FALSE, "Identifier"="RSCMXPGPRF_ATTR_HIDDEN_POWER_MEASUREMENT_LIMIT_CHECK_RESULT_LIST_MINIMUM_PEAK", "Descriptive Name"="Power Measurement Limit Check Result List Minimum Peak", "Data Type"=6, "Command"="CALC:GPRF:MEAS{instance}:POW:LIST:PEAK:MIN?", "Access"=0, "Range Table"="", "Read Callback"="", "Write Callback"="", "Supported Models"="", "Instrument Options"="", "Flags"=8, "Help"="Returns power results for segment <ListIndex>, see Results in List Mode.\n\nAvailable Repeated Capabilities:\ninstance: i0, i1, i2, i3, i4, i5, i6, i7, i8, i9, i10, i11, i12, i13, i14, i15, i16, i17, i18, i19, i20, i21, i22, i23, i24, i25, i26, i27, i28, i29, i30, i31, i32\r\n\nRemote-control command(s):\nCALCulate:GPRF:MEAS<i>:POWer:LIST:PEAK:MINimum?"}, {"Level"=3, "Class Only"=FALSE, "Identifier"="RSCMXPGPRF_ATTR_HIDDEN_READ_POWER_MEASUREMENT_STANDARD_DEVIATION_LIST_MODE", "Descriptive Name"="Read Power Measurement Standard Deviation List Mode", "Data Type"=2, "Command"="READ:GPRF:MEAS{instance}:POW:LIST:SDEV?", "Access"=0, "Range Table"="", "Read Callback"="", "Write Callback"="", "Supported Models"="", "Instrument Options"="", "Flags"=8, "Help"="Returns power results for segment <ListIndex>, see Results in List Mode.\n\nAvailable Repeated Capabilities:\ninstance: i0, i1, i2, i3, i4, i5, i6, i7, i8, i9, i10, i11, i12, i13, i14, i15, i16, i17, i18, i19, i20, i21, i22, i23, i24, i25, i26, i27, i28, i29, i30, i31, i32\r\n\nRemote-control command(s):\nREAD:GPRF:MEAS<i>:POWer:LIST:SDEViation?"}, {"Level"=3, "Class Only"=FALSE, "Identifier"="RSCMXPGPRF_ATTR_HIDDEN_FETCH_POWER_MEASUREMENT_STANDARD_DEVIATION_LIST_MODE", "Descriptive Name"="Fetch Power Measurement Standard Deviation List Mode", "Data Type"=2, "Command"="FETCh:GPRF:MEAS{instance}:POW:LIST:SDEV?", "Access"=0, "Range Table"="", "Read Callback"="", "Write Callback"="", "Supported Models"="", "Instrument Options"="", "Flags"=8, "Help"="Returns power results for segment <ListIndex>, see Results in List Mode.\n\nAvailable Repeated Capabilities:\ninstance: i0, i1, i2, i3, i4, i5, i6, i7, i8, i9, i10, i11, i12, i13, i14, i15, i16, i17, i18, i19, i20, i21, i22, i23, i24, i25, i26, i27, i28, i29, i30, i31, i32\r\n\nRemote-control command(s):\nFETCh:GPRF:MEAS<i>:POWer:LIST:SDEViation?"}, {"Level"=3, "Class Only"=FALSE, "Identifier"="RSCMXPGPRF_ATTR_FETCH_POWER_MEASUREMENT_STATISTICS_TRACE_APD", "Descriptive Name"="Fetch Power Measurement Statistics Trace APD", "Data Type"=6, "Command"="FETC:GPRF:MEAS{instance}:POW:APD?", "Access"=0, "Range Table"="", "Read Callback"="", "Write Callback"="", "Supported Models"="", "Instrument Options"="", "Flags"=0, "Help"="Returns the APD diagram contents.\n\nAvailable Repeated Capabilities:\ninstance: i0, i1, i2, i3, i4, i5, i6, i7, i8, i9, i10, i11, i12, i13, i14, i15, i16, i17, i18, i19, i20, i21, i22, i23, i24, i25, i26, i27, i28, i29, i30, i31, i32\r\n\nRemote-control command(s):\nFETCh:GPRF:MEAS<i>:POWer:APD?"}, {"Level"=3, "Class Only"=FALSE, "Identifier"="RSCMXPGPRF_ATTR_FETCH_POWER_MEASUREMENT_STATISTICS_TRACE_CCDF", "Descriptive Name"="Fetch Power Measurement Statistics Trace CCDF", "Data Type"=6, "Command"="FETC:GPRF:MEAS{instance}:POW:CCDF?", "Access"=0, "Range Table"="", "Read Callback"="", "Write Callback"="", "Supported Models"="", "Instrument Options"="", "Flags"=0, "Help"="Returns the CCDF diagram contents.\n\nAvailable Repeated Capabilities:\ninstance: i0, i1, i2, i3, i4, i5, i6, i7, i8, i9, i10, i11, i12, i13, i14, i15, i16, i17, i18, i19, i20, i21, i22, i23, i24, i25, i26, i27, i28, i29, i30, i31, i32\r\n\nRemote-control command(s):\nFETCh:GPRF:MEAS<i>:POWer:CCDF?"}, {"Level"=3, "Class Only"=FALSE, "Identifier"="RSCMXPGPRF_ATTR_FETCH_POWER_MEASUREMENT_CCDF_PERCENTILES", "Descriptive Name"="Fetch Power Measurement CCDF Percentiles", "Data Type"=6, "Command"="FETC:GPRF:MEAS{instance}:POW:CCDF:PROB?", "Access"=0, "Range Table"="", "Read Callback"="", "Write Callback"="", "Supported Models"="", "Instrument Options"="", "Flags"=0, "Help"="Returns power values with a certain probability, taken from the CCDF diagram.\n\nAvailable Repeated Capabilities:\ninstance: i0, i1, i2, i3, i4, i5, i6, i7, i8, i9, i10, i11, i12, i13, i14, i15, i16, i17, i18, i19, i20, i21, i22, i23, i24, i25, i26, i27, i28, i29, i30, i31, i32\r\n\nRemote-control command(s):\nFETCh:GPRF:MEAS<i>:POWer:CCDF:PROBability?"}, {"Level"=3, "Class Only"=FALSE, "Identifier"="RSCMXPGPRF_ATTR_FETCH_POWER_MEASUREMENT_CCDF_STATISTIC_RESULTS", "Descriptive Name"="Fetch Power Measurement CCDF Statistic Results", "Data Type"=6, "Command"="FETC:GPRF:MEAS{instance}:POW:CCDF:POW?", "Access"=0, "Range Table"="", "Read Callback"="", "Write Callback"="", "Supported Models"="", "Instrument Options"="", "Flags"=0, "Help"="Returns some statistic results for the power samples.\n\nAvailable Repeated Capabilities:\ninstance: i0, i1, i2, i3, i4, i5, i6, i7, i8, i9, i10, i11, i12, i13, i14, i15, i16, i17, i18, i19, i20, i21, i22, i23, i24, i25, i26, i27, i28, i29, i30, i31, i32\r\n\nRemote-control command(s):\nFETCh:GPRF:MEAS<i>:POWer:CCDF:POWer?"}, {"Level"=3, "Class Only"=FALSE, "Identifier"="RSCMXPGPRF_ATTR_FETCH_POWER_MEASUREMENT_SAMPLE_STATISTIC_COUNTERS", "Descriptive Name"="Fetch Power Measurement Sample Statistic Counters", "Data Type"=6, "Command"="FETC:GPRF:MEAS{instance}:POW:CCDF:SAMP?", "Access"=0, "Range Table"="", "Read Callback"="", "Write Callback"="", "Supported Models"="", "Instrument Options"="", "Flags"=0, "Help"="Returns the sample counters for the APD and CCDF results.\n\nAvailable Repeated Capabilities:\ninstance: i0, i1, i2, i3, i4, i5, i6, i7, i8, i9, i10, i11, i12, i13, i14, i15, i16, i17, i18, i19, i20, i21, i22, i23, i24, i25, i26, i27, i28, i29, i30, i31, i32\r\n\nRemote-control command(s):\nFETCh:GPRF:MEAS<i>:POWer:CCDF:SAMPle?"}, {"Level"=1, "Class Only"=TRUE, "Identifier"="", "Descriptive Name"="IQ vs Slot Measurement", "Data Type"=0, "Command"="", "Access"=0, "Range Table"="", "Read Callback"="", "Write Callback"="", "Supported Models"="", "Instrument Options"="", "Flags"=0, "Help"="IQ vs Slot measurement configuration and control."}, {"Level"=2, "Class Only"=TRUE, "Identifier"="", "Descriptive Name"="Configuration", "Data Type"=0, "Command"="", "Access"=0, "Range Table"="", "Read Callback"="", "Write Callback"="", "Supported Models"="", "Instrument Options"="", "Flags"=0, "Help"="Configuration of IQ vs Slot measurement."}, {"Level"=3, "Class Only"=FALSE, "Identifier"="RSCMXPGPRF_ATTR_IQ_VS_SLOT_MEASUREMENT_STEP_LENGTH", "Descriptive Name"="IQ vs Slot Measurement Step Length", "Data Type"=1, "Command"="CONF:GPRF:MEAS{instance}:IQVS:SLEN", "Access"=2, "Range Table"="rsCmxpGprf_rngIqvsStepLength", "Read Callback"="", "Write Callback"="", "Supported Models"="", "Instrument Options"="", "Flags"=0, "Help"="Selects the time between the beginning of two consecutive measurement steps.\n\nAvailable Repeated Capabilities:\ninstance: i0, i1, i2, i3, i4, i5, i6, i7, i8, i9, i10, i11, i12, i13, i14, i15, i16, i17, i18, i19, i20, i21, i22, i23, i24, i25, i26, i27, i28, i29, i30, i31, i32\r\n\nRemote-control command(s):\nCONFigure:GPRF:MEAS<i>:IQVSlot:SLENgth"}, {"Level"=3, "Class Only"=FALSE, "Identifier"="RSCMXPGPRF_ATTR_IQ_VS_SLOT_MEASUREMENT_MEASUREMENT_LENGTH", "Descriptive Name"="IQ vs Slot Measurement Measurement Length", "Data Type"=1, "Command"="CONF:GPRF:MEAS{instance}:IQVS:MLEN", "Access"=2, "Range Table"="", "Read Callback"="", "Write Callback"="", "Supported Models"="", "Instrument Options"="", "Flags"=0, "Help"="Selects the length of the averaging intervals that the R&S CMW uses to calculate the &apos;I/Q vs. Slot&apos; results for each measurement step.\n\nAvailable Repeated Capabilities:\ninstance: i0, i1, i2, i3, i4, i5, i6, i7, i8, i9, i10, i11, i12, i13, i14, i15, i16, i17, i18, i19, i20, i21, i22, i23, i24, i25, i26, i27, i28, i29, i30, i31, i32\r\n\nRemote-control command(s):\nCONFigure:GPRF:MEAS<i>:IQVSlot:MLENgth"}, {"Level"=3, "Class Only"=FALSE, "Identifier"="RSCMXPGPRF_ATTR_IQ_VS_SLOT_MEASUREMENT_FREQUENCY_ERROR_LIMIT", "Descriptive Name"="IQ vs Slot Measurement Frequency Error Limit", "Data Type"=1, "Command"="CONF:GPRF:MEAS{instance}:IQVS:FEL", "Access"=2, "Range Table"="rsCmxpGprf_rngIqvsFELimit", "Read Callback"="", "Write Callback"="", "Supported Models"="", "Instrument Options"="", "Flags"=0, "Help"="Defines a minimum average signal level relative to the &apos;Expected Nominal Power&apos; for all measurement steps to be considered for the calculation of the average frequency per subsweep and the &apos;Overall Frequency Error&apos;.\n\nAvailable Repeated Capabilities:\ninstance: i0, i1, i2, i3, i4, i5, i6, i7, i8, i9, i10, i11, i12, i13, i14, i15, i16, i17, i18, i19, i20, i21, i22, i23, i24, i25, i26, i27, i28, i29, i30, i31, i32\r\n\nRemote-control command(s):\nCONFigure:GPRF:MEAS<i>:IQVSlot:FELimit"}, {"Level"=3, "Class Only"=FALSE, "Identifier"="RSCMXPGPRF_ATTR_IQ_VS_SLOT_MEASUREMENT_REPETITION_MODE", "Descriptive Name"="IQ vs Slot Measurement Repetition Mode", "Data Type"=0, "Command"="CONF:GPRF:MEAS{instance}:IQVS:REP", "Access"=2, "Range Table"="rsCmxpGprf_rngRepMode", "Read Callback"="", "Write Callback"="", "Supported Models"="", "Instrument Options"="", "Flags"=0, "Help"="Specifies the repetition mode of the measurement; see Statistical Settings. The repetition mode specifies whether the measurement is stopped after a single shot or repeated continuously.\n\nAvailable Repeated Capabilities:\ninstance: i0, i1, i2, i3, i4, i5, i6, i7, i8, i9, i10, i11, i12, i13, i14, i15, i16, i17, i18, i19, i20, i21, i22, i23, i24, i25, i26, i27, i28, i29, i30, i31, i32\r\n\nRemote-control command(s):\nCONFigure:GPRF:MEAS<i>:IQVSlot:REPetition"}, {"Level"=3, "Class Only"=FALSE, "Identifier"="RSCMXPGPRF_ATTR_IQ_VS_SLOT_MEASUREMENT_COUNT", "Descriptive Name"="IQ vs Slot Measurement Count", "Data Type"=0, "Command"="CONF:GPRF:MEAS{instance}:IQVS:SCO", "Access"=2, "Range Table"="rsCmxpGprf_rngIqvsCount", "Read Callback"="", "Write Callback"="", "Supported Models"="", "Instrument Options"="", "Flags"=0, "Help"="Specifies the statistic count of the measurement; see Statistical Settings. The statistic count is equal to the number of measurement intervals per single shot.\n\nAvailable Repeated Capabilities:\ninstance: i0, i1, i2, i3, i4, i5, i6, i7, i8, i9, i10, i11, i12, i13, i14, i15, i16, i17, i18, i19, i20, i21, i22, i23, i24, i25, i26, i27, i28, i29, i30, i31, i32\r\n\nRemote-control command(s):\nCONFigure:GPRF:MEAS<i>:IQVSlot:SCOunt"}, {"Level"=3, "Class Only"=FALSE, "Identifier"="RSCMXPGPRF_ATTR_IQ_VS_SLOT_MEASUREMENT_FILTER_TYPE", "Descriptive Name"="IQ vs Slot Measurement Filter Type", "Data Type"=0, "Command"="CONF:GPRF:MEAS{instance}:IQVS:FTYP", "Access"=2, "Range Table"="rsCmxpGprf_rngIqvsFilterType", "Read Callback"="", "Write Callback"="", "Supported Models"="", "Instrument Options"="", "Flags"=0, "Help"="Selects the IF filter type.\n\nAvailable Repeated Capabilities:\ninstance: i0, i1, i2, i3, i4, i5, i6, i7, i8, i9, i10, i11, i12, i13, i14, i15, i16, i17, i18, i19, i20, i21, i22, i23, i24, i25, i26, i27, i28, i29, i30, i31, i32\r\n\nRemote-control command(s):\nCONFigure:GPRF:MEAS<i>:IQVSlot:FTYPe"}, {"Level"=3, "Class Only"=FALSE, "Identifier"="RSCMXPGPRF_ATTR_IQ_VS_SLOT_MEASUREMENT_TRIGGER_SOURCE", "Descriptive Name"="IQ vs Slot Measurement 
